vi "9759 RevB Core.vi"(4 "dt (s)":sgl, 6 "Device Inputs in":dbl[](array[numeric]), 8 "error in (no error)":errorcluster, 9 "Device Outputs in":dbl[](array[numeric]), 10 "9759 RevB in":T1 {"Settings"."ControlCals"."ThetaLH (deg)" format="%.3f"; "Settings"."ControlCals"."ULHLag (sec)" format="%.3f"; "Settings"."ControlCals"."USLag (sec)" format="%.3f"; "Settings"."ControlCals"."TLead (sec)" format="%.3f"; "Settings"."ControlCals"."TLag (sec)" format="%.3f"}, 11 "FPGA Ref in":T2) -> (0 "error out":errorcluster, 1 "Device Outputs out":dbl[](array[numeric]), 2 "9759 RevB out":T1 {"Settings"."ControlCals"."ThetaLH (deg)" format="%.3f"; "Settings"."ControlCals"."ULHLag (sec)" format="%.3f"; "Settings"."ControlCals"."USLag (sec)" format="%.3f"; "Settings"."ControlCals"."TLead (sec)" format="%.3f"; "Settings"."ControlCals"."TLag (sec)" format="%.3f"}, 3 "FPGA Ref out":T2)   [LabVIEW 2015, in "NI 9759 RevB Custom Device.lvlib"]
uses:
  NI 9759 RevB Custom Device.lvlib
  Shared/Types/9759 RevB FPGA Ref.ctl
  Shared/Types/9759 RevB.ctl
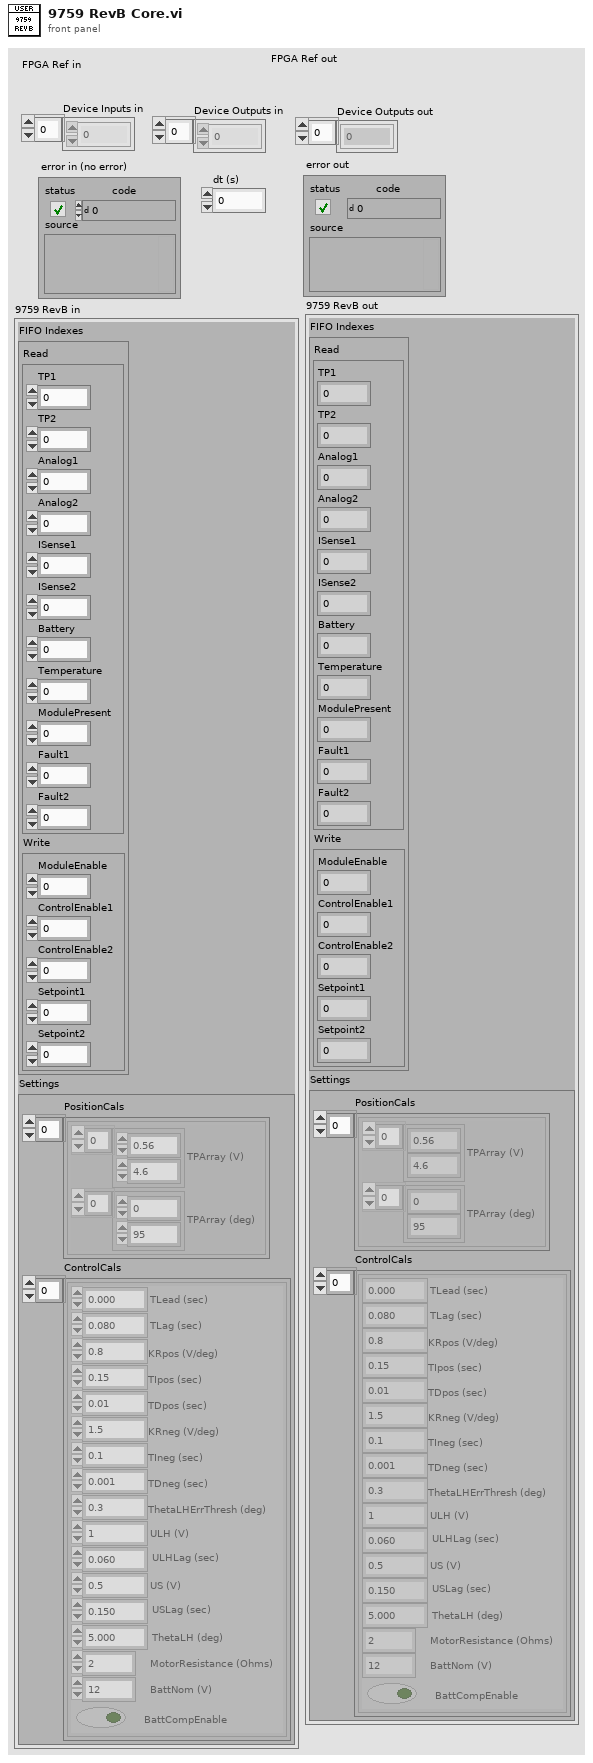
[diagram p1: front panel]
types:
  T1 = typedef "NI 9759 RevB Custom Device.lvlib/9759 RevB.ctl" = cluster{"FIFO Indexes":cluster{"Read":cluster{"TP1":i32, "TP2":i32, "Analog1":i32, "Analog2":i32, "ISense1":i32, "ISense2":i32, "Battery":i32, "Temperature":i32, "ModulePresent":i32, "Fault1":i32, "Fault2":i32}, "Write":cluster{"ModuleEnable":i32, "ControlEnable1":i32, "ControlEnable2":i32, "Setpoint1":i32, "Setpoint2":i32}}, "Settings":cluster{"PositionCals":cluster{"TPArray (V)":sgl[], "TPArray (deg)":sgl[]}[], "ControlCals":cluster{"TLead (sec)":sgl, "TLag (sec)":sgl, "KRpos (V/deg)":sgl, "TIpos (sec)":sgl, "TDpos (sec)":sgl, "KRneg (V/deg)":sgl, "TIneg (sec)":sgl, "TDneg (sec)":sgl, "ThetaLHErrThresh (deg)":sgl, "ULH (V)":sgl, "ULHLag (sec)":sgl, "US (V)":sgl, "USLag (sec)":sgl, "ThetaLH (deg)":sgl, "MotorResistance (Ohms)":sgl, "BattNom (V)":sgl, "BattCompEnable":bool}[]}}
  T2 = typedef "NI 9759 RevB Custom Device.lvlib/9759 RevB FPGA Ref.ctl" = refnum<k20>
  T3 = cluster{"TP1":i32, "TP2":i32, "Analog1":i32, "Analog2":i32, "ISense1":i32, "ISense2":i32, "Battery":i32, "Temperature":i32, "ModulePresent":i32, "Fault1":i32, "Fault2":i32}
  T4 = cluster{"ModuleEnable":i32, "ControlEnable1":i32, "ControlEnable2":i32, "Setpoint1":i32, "Setpoint2":i32}
  T5 = cluster{"TPArray (V)":sgl[], "TPArray (deg)":sgl[]}[]
  T6 = cluster{"TLead (sec)":sgl, "TLag (sec)":sgl, "KRpos (V/deg)":sgl, "TIpos (sec)":sgl, "TDpos (sec)":sgl, "KRneg (V/deg)":sgl, "TIneg (sec)":sgl, "TDneg (sec)":sgl, "ThetaLHErrThresh (deg)":sgl, "ULH (V)":sgl, "ULHLag (sec)":sgl, "US (V)":sgl, "USLag (sec)":sgl, "ThetaLH (deg)":sgl, "MotorResistance (Ohms)":sgl, "BattNom (V)":sgl, "BattCompEnable":bool}[]
  T7 = cluster{"TP1":sgl, "TP2":sgl, "Temperature":sgl, "Battery":sgl, "ModulePresent":bool}
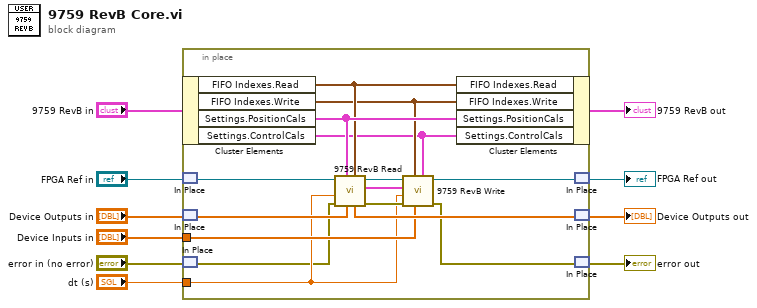
[diagram p0: block diagram]
diagram:
  n1 = in-place {
    in-place-border: "Device Inputs in" -> [w16]
    in-place-border: "dt (s)" -> [w13]
    n2 = in-place-cluster #1("9759 RevB in") -> ("FIFO Indexes.Read"=w21:T3, "FIFO Indexes.Write"=w15:T4, "Settings.PositionCals"=w22:T5, "Settings.ControlCals"=w14:T6)
    n3 = in-place-match #2("FPGA Ref in") -> (w25:T2)
    n4 = in-place-match #3("Device Outputs in") -> (w24:dbl[])
    n5 = in-place-match #4("error in (no error)") -> (w12:errorcluster)
    n6 = call "9759 RevB Read.vi"("FIFO Indexes.Read"=w21, "Device Outputs in"=w24, "Settings.PositionCals"=w22, "error in"=w12, "dt (sec)"=w13, "FPGA Ref in"=w25) -> ("error out"=w18:errorcluster, "Data"=w17:T7, "FPGA Ref out"=w20:T2, "Device Outputs out"=w23:dbl[])  [unwired: 2 in]
    n7 = call "9759 RevB Write.vi"("Settings.ControlCals"=w14, "Device Inputs"=w16, "FIFO Indexes.Write"=w15, "error in"=w18, "dt (sec)"=w13, "Data"=w17, "FPGA Ref in"=w20) -> ("error out"=w11:errorcluster, "FPGA Ref out"=w19:T2)  [unwired: 3 in]
    n8 = in-place-cluster #1("FIFO Indexes.Read"=w21, "FIFO Indexes.Write"=w15, "Settings.PositionCals"=w22, "Settings.ControlCals"=w14) -> (→"9759 RevB out":T1)
    n9 = in-place-match #2(w19) -> (→"FPGA Ref out":T2)
    n10 = in-place-match #3(w23) -> (→"Device Outputs out":dbl[])
    n11 = in-place-match #4(w11) -> (→"error out":errorcluster)
  }
